vi "Serial Port Test.vi"() -> ()   [LabVIEW 2015]
uses:
  Libraries/RDS Serial Handler/RDS Serial Instrument.lvclass
  Libraries/RDS Serial Handler/RDS Serial Instrument.lvclass/RDS Serial Instrument.ctl
panel:
  in  "Disconnect":bool
  in  "Send Data":bool
  out "Read String":string
  in  "Termination Char(s)":string
  in  "baud rate (9600)":u32=9600
  in  "VISA resource name":refnum<visa-resource-name>="COM1"
  in  "Init Port":bool
  out "Connected":bool
  in  "stop":bool
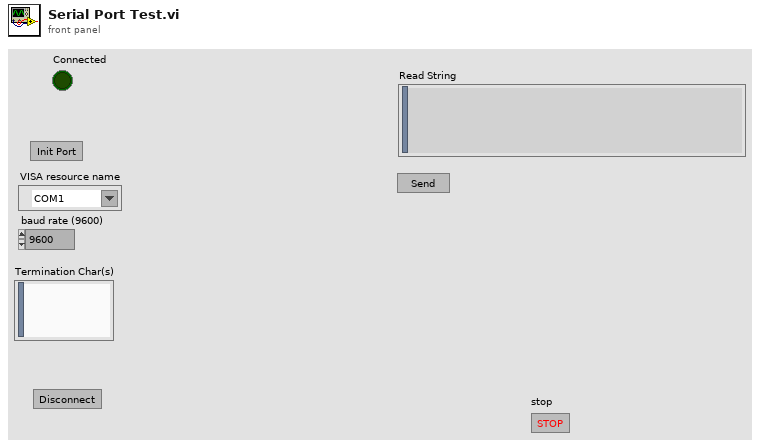
[diagram p1: front panel]
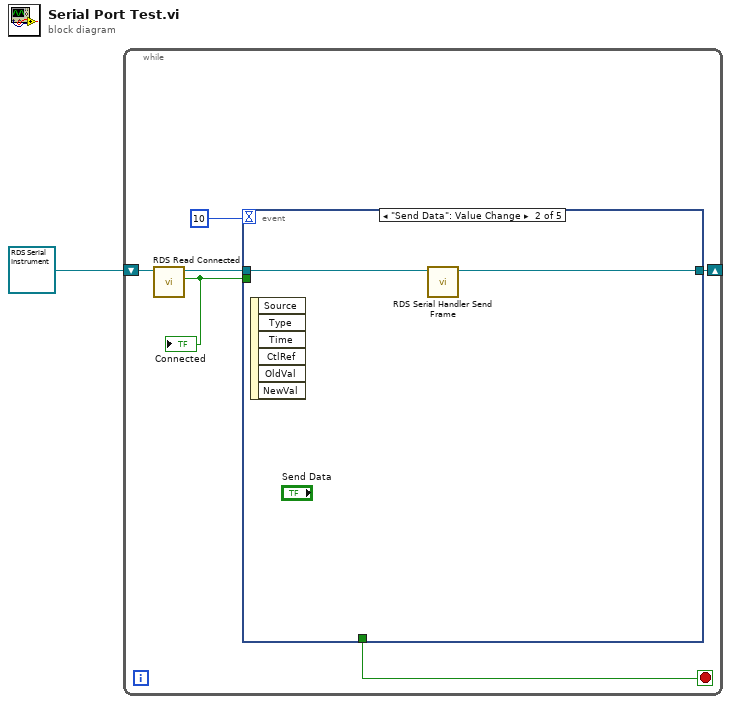
[diagram p0: block diagram]
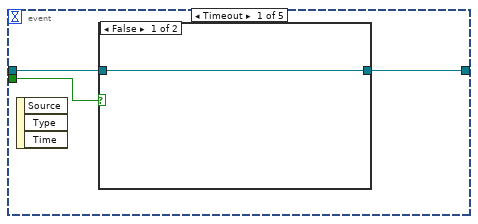
[diagram p2: hidden frame]
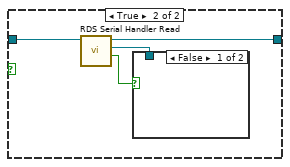
[diagram p3: hidden frame]
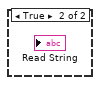
[diagram p4: hidden frame]
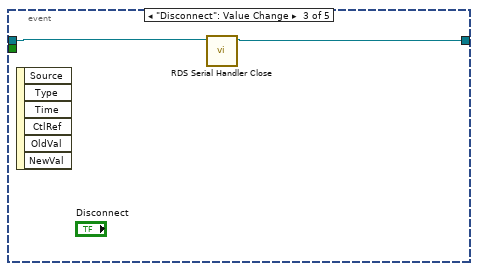
[diagram p5: hidden frame]
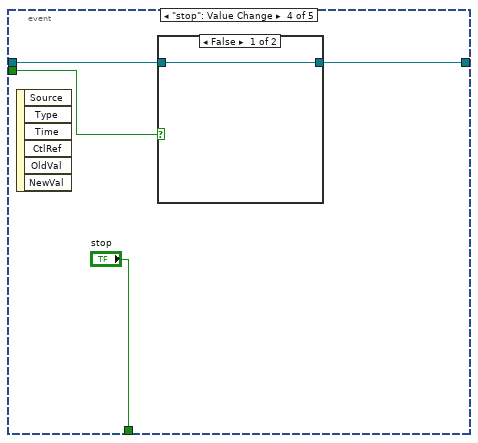
[diagram p6: hidden frame]
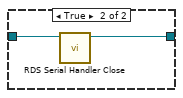
[diagram p7: hidden frame]
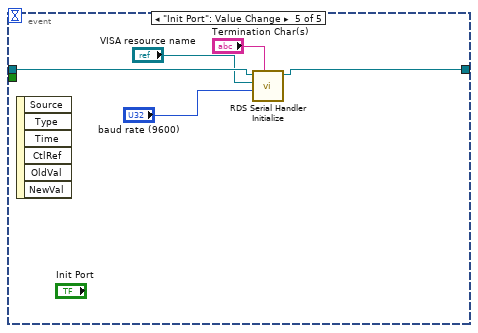
[diagram p8: hidden frame]
diagram:
  n1 = while {
    shift-right: [w4] -> _
    shift-left: refnum<class "RDS Serial Instrument.lvclass"> refnum ("RDS Instrument") -> [w7]
    stop <- w3 stop-if-true
    n2 = call "RDS Read Connected.vi"("RDS Serial Instrument in"=w7) -> ("Connected"=w5:bool, "RDS Serial Instrument out"=w6:refnum<class "RDS Serial Instrument.lvclass">)  [unwired: 8 in, 1 out]
    "Connected" <- w5
    n3 = event shown="[1] \"Send Data\": Value Change" {
      selector: _ -> [_ _ _ _ _]
      dyn-events: _ -> [_ _ _ _ _]
      timeout: 10 -> [_ _ _ _ _]
      tunnel: w6 -> [w10 w17 w19 w22 w31]
      tunnel: w5 -> [w8 _ _ w23 _]
      tunnel: [w9 w16 w18 w21 w28] -> w4
      tunnel: [_ _ _ "stop" _] -> w3
      event Timeout {
        n4 = event-data() -> ()  [unwired: 1 in, 3 out]
        n5 = case shown="False" w8 {
          tunnel: w10 -> [w11 w15]
          tunnel: [w11 w14] -> w9
          frame False {
          }
          frame True {
            n6 = call "RDS Serial Handler Read.vi"("RDS Serial Instrument in"=w15) -> ("Data Valid?"=w12:bool, "RDS Serial Frame out"=w13:refnum<class "RDS Serial Frame.lvclass">, "RDS Serial Instrument out"=w14:refnum<class "RDS Serial Instrument.lvclass">)  [unwired: 7 in, 1 out]
            n7 = case shown="False" w12 {
              tunnel: w13 -> [_ _]
              frame False {
              }
              frame True {
              }
            }
          }
        }
      }
      event "Send Data": Value Change {
        n8 = event-data() -> ()  [unwired: 1 in, 6 out]
        n9 = call "RDS Serial Handler Send Frame.vi"("RDS Serial Instrument in"=w17) -> ("RDS Serial Instrument out"=w16:refnum<class "RDS Serial Instrument.lvclass">)  [unwired: 9 in, 1 out]
      }
      event "Disconnect": Value Change {
        n10 = event-data() -> ()  [unwired: 1 in, 6 out]
        n11 = call "RDS Serial Handler Close.vi"("RDS Serial Instrument in"=w19) -> ("RDS Serial Instrument out"=w18:refnum<class "RDS Serial Instrument.lvclass">)  [unwired: 9 in, 1 out]
      }
      event "stop": Value Change {
        n12 = event-data() -> ()  [unwired: 1 in, 6 out]
        n13 = case shown="False" w23 {
          tunnel: w22 -> [w24 w26]
          tunnel: [w24 w25] -> w21
          frame False {
          }
          frame True {
            n14 = call "RDS Serial Handler Close.vi"("RDS Serial Instrument in"=w26) -> ("RDS Serial Instrument out"=w25:refnum<class "RDS Serial Instrument.lvclass">)  [unwired: 9 in, 1 out]
          }
        }
      }
      event "Init Port": Value Change {
        n15 = event-data() -> ()  [unwired: 1 in, 6 out]
        n16 = call "RDS Serial Handler Initialize.vi"("Termination Char(s)"="Termination Char(s)", "baud rate (9600)"="baud rate (9600)", "VISA resource name"="VISA resource name", "RDS Serial Instrument in"=w31) -> ("RDS Serial Instrument out"=w28:refnum<class "RDS Serial Instrument.lvclass">)  [unwired: 6 in, 1 out]
      }
    }
  }
